vi "Log_display.vi"() -> ()   [LabVIEW 2017]
panel:
  in  "stop":bool
  out "log":string
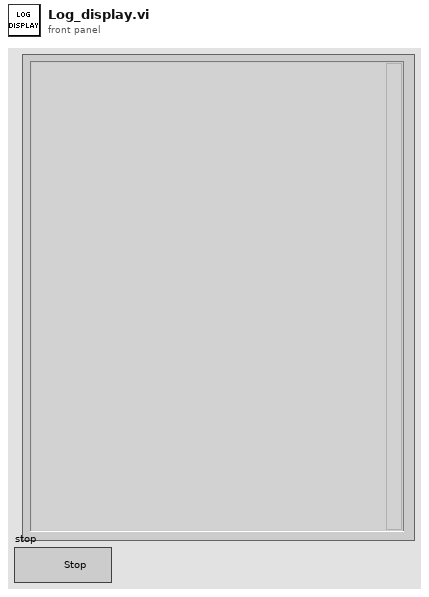
[diagram p1: front panel]
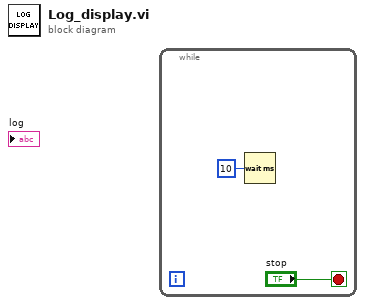
[diagram p0: block diagram]
diagram:
  n1 = while {
    stop <- "stop" stop-if-true
    n2 = Wait (ms)(milliseconds to wait=u32 10) -> ()  [unwired: 1 out]
  }
